vi "02 Setting a servo.vi"() -> ()   [LabVIEW 2019]
uses:
  <vilib>/Instr/_visa.llb/VISA Configure Serial Port (Instr).vi
panel:
  out "position read":u8=100
  in  "Position":u8(slide)=98 scale=0.0..180.0
  in  "MicroPython code":string="'''\nhttps://docs.micropython.org/en/latest/pyboard/tutorial/servo.html\n     \nconnections: \nGround (B) - GND \nPower  (R)   - 3V3 \nNC\nSignal -  pin X1\n'''\n\nimport pyb\n\nservo1 = pyb.Servo(1)   # pix X1\n\n#set the angle\nservo1.angle(45)\n"
  in  "stop":bool
  out "Connected":bool
  in  "MicroPython Port":refnum<visa-resource-name>="ASRL26::INSTR"
  # "Download and run the MicroPython  Code  below\n\nSelect the board port below\n\nHit the Run arrow and move the position slider - does the servo move?"
  # "Hit Cmd E to see the diagram (code)"
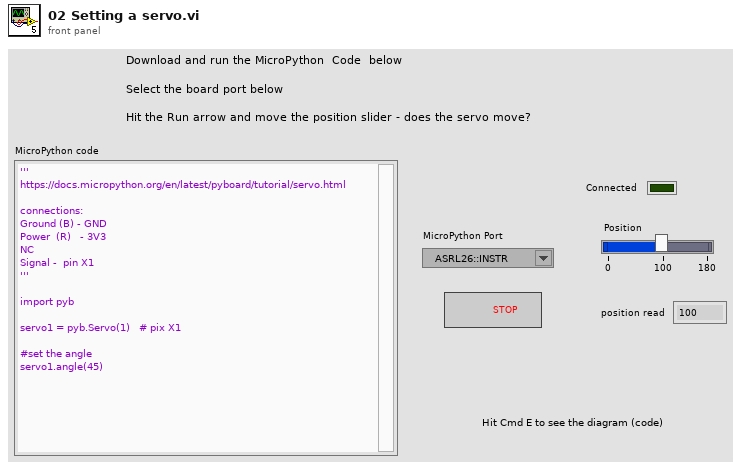
[diagram p1: front panel]
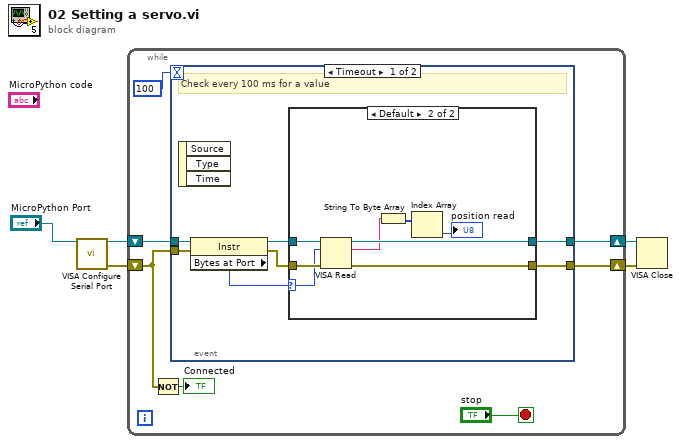
[diagram p0: block diagram]
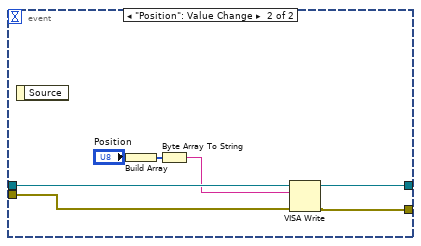
[diagram p3: hidden frame]
diagram:
  n1 = call-poly "VISA Configure Serial Port"("VISA resource name"="MicroPython Port") -> ("VISA resource name out"=w4:refnum<visa-resource-name>, "error out"=w3:errorcluster)  [unwired: 13 in]
  n2 = while {
    shift-right: [w10] -> w1
    shift-left: w4 -> [w12]
    shift-right: [w11] -> w2
    shift-left: w3 -> [w8]
    stop <- "stop" stop-if-true
    n3 = Not(x=w8) -> (.not. x?=→"Connected":bool)
    n4 = event shown="[0] Timeout" {
      selector: _ -> [_ _]
      dyn-events: _ -> [_ _]
      timeout: 100 -> [_ _]
      tunnel: w12 -> [w19 w36]
      tunnel: [w16 w34] -> w11
      tunnel: [w15 w33] -> w10
      tunnel: w8 -> [w13 w35]
      event Timeout {
        # "Check every 100 ms for a value"
        n5 = event-data() -> ()  [unwired: 1 in, 3 out]
        n6 = property class="Instr"(reference=w19, error in=w13) -> (reference out=w18:refnum<visa-resource-name>, error out=w17:errorcluster, "Bytes at Port"=w14:u32)
        n7 = case shown="Default" w14 {
          selector: w14 -> [_ w25]
          tunnel: w18 -> [w21 w29]
          tunnel: w17 -> [w20 w28]
          tunnel: [w20 w27] -> w16
          tunnel: [w21 w26] -> w15
          frame 0 {
          }
          frame Default {
            n8 = VISA Read(VISA resource name=w29, byte count=w25, error in (no error)=w28) -> (VISA resource name out=w26:refnum<visa-resource-name>, read buffer=w24:string, error out=w27:errorcluster)  [unwired: 1 out]
            n9 = String To Byte Array(string=w24) -> (unsigned byte array=w23:u8[])
            n10 = Index Array(array=w23) -> (element=→"position read":u8)  [unwired: 1 in]
          }
        }
      }
      event "Position": Value Change {
        n11 = event-data() -> ()  [unwired: 1 in, 1 out]
        n12 = Build Array("Position") -> (w31:u8[])
        n13 = Byte Array To String(unsigned byte array=w31) -> (string=w30:string)
        n14 = VISA Write(VISA resource name=w36, write buffer=w30, error in (no error)=w35) -> (VISA resource name out=w33:refnum<visa-resource-name>, error out=w34:errorcluster)  [unwired: 1 out]
      }
    }
  }
  n15 = VISA Close(VISA resource name=w1, error in (no error)=w2) -> ()  [unwired: 1 out]
